vi "Banana Factory.vi"(6 "Strategies.Test":T1, 8 "Clear":bool, 9 "Strategies.Assert":T2, 10 "Peels":refnum<class "BananaPeel.lvclass">[](array[class]), 11 "Variety":string) -> (2 "Bunch":refnum<class "Banana.lvclass">, 3 "Variety Configured":string)   [LabVIEW 2021, in "Bananas.lvlib" / "Banana.lvclass"]
uses:
  Banana.lvclass
  BananaPeel/BananaPeel.lvclass
  Assertion Strategies -- cluster.ctl
  AssertTrue/AssertTrue.lvclass
  AssertFalse/AssertFalse.lvclass
  Test Strategies -- cluster.ctl
  DefineTest/DefineTest.lvclass
  Banana.lvclass/Banana.ctl
  Bananas.lvlib
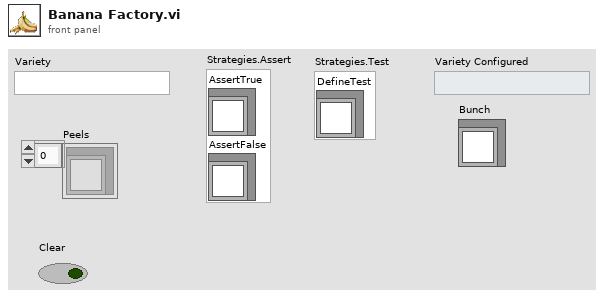
[diagram p1: front panel]
types:
  T1 = typedef "Bananas.lvlib/Test Strategies -- cluster.ctl" = cluster{"DefineTest":refnum<class "DefineTest.lvclass">}
  T2 = typedef "Bananas.lvlib/Assertion Strategies -- cluster.ctl" = cluster{"AssertTrue":refnum<class "AssertTrue.lvclass">, "AssertFalse":refnum<class "AssertFalse.lvclass">}
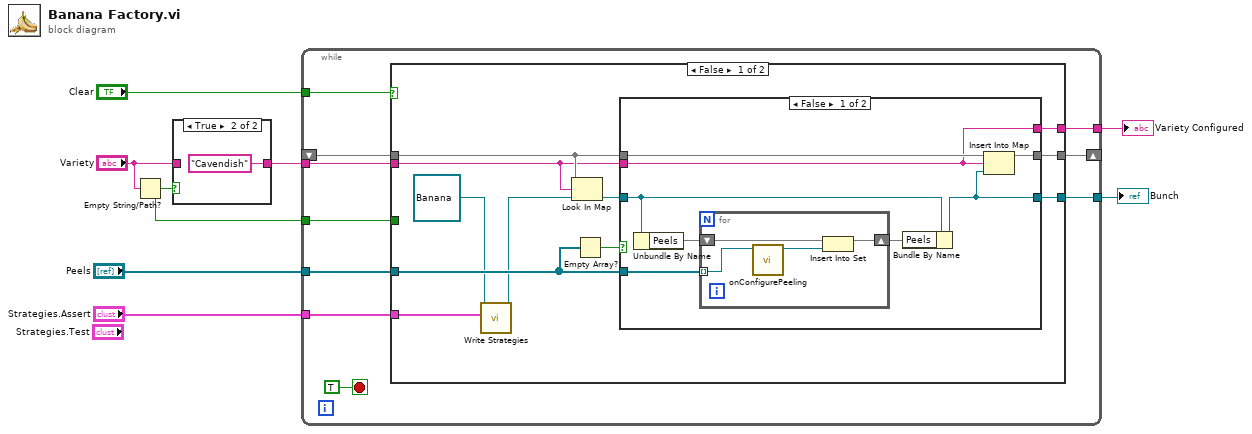
[diagram p0: block diagram]
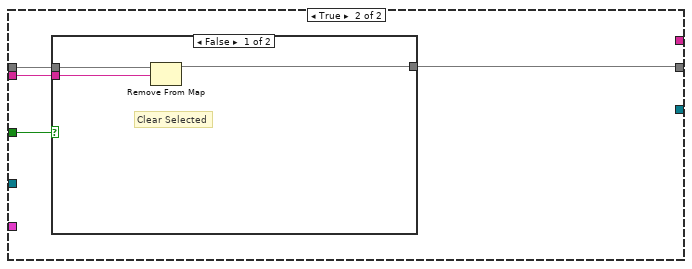
[diagram p4: hidden frame]
diagram:
  n1 = Empty String/Path?(string/path="Variety") -> (empty?=w2:bool)
  n2 = case shown="True" w2 {
    tunnel: [w9 "Cavendish" ("Variety")] -> w7
    tunnel: "Variety" -> [w9 _]
    frame False {
    }
    frame True {
    }
  }
  n3 = while {
    shift-right: [w18] -> _
    shift-left: _ -> [w19]
    tunnel: w7 -> [w16]
    tunnel: [w17] -> w8
    tunnel: "Peels" -> [w15]
    tunnel: "Strategies.Assert" -> [w14]
    tunnel: "Clear" -> [w13]
    tunnel: w2 -> [w12]
    tunnel: [w11] -> w1
    stop <- TRUE stop-if-true
    n4 = case shown="False" w13 {
      tunnel: w19 -> [w31 w49]
      tunnel: [w30 w47] -> w18
      tunnel: [w28 _] -> w17
      tunnel: w16 -> [w27 w48]
      tunnel: w15 -> [w26 _]
      tunnel: w14 -> [w22 _]
      tunnel: w12 -> [_ w50]
      tunnel: [w21 _] -> w11
      frame False {
        n5 = call "Write Strategies.vi"("Strategies.Assert"=w22, "Banana in"=refnum<class "Banana.lvclass"> refnum ("Banana")) -> ("Banana out"=w23:refnum<class "Banana.lvclass">)  [unwired: 9 in]
        n6 = Look In Map(map=w31, key=w27, default value=w23) -> (value=w29:refnum<class "Banana.lvclass">)  [unwired: 1 out]
        n7 = Empty Array?(array=w26) -> (empty?=w25:bool)
        n8 = case shown="False" w25 {
          tunnel: w31 -> [w39 w46]
          tunnel: [w38 w46] -> w30
          tunnel: w29 -> [w34 w45]
          tunnel: [w35 w45] -> w28
          tunnel: w27 -> [w32 w44]
          tunnel: w26 -> [w33 _]
          tunnel: [w32 w44] -> w21
          frame False {
            n9 = Unbundle By Name(w34) -> ("Peels"=w37:set{refnum<class "BananaPeel.lvclass">})
            n10 = for {
              shift-right: [w42] -> w36
              shift-left: w37 -> [w43]
              tunnel: w33 -> [w40] mode=indexing
              n11 = call-dynamic "onConfigurePeeling.vi"("BananaPeel in"=w40) -> ("BananaPeel out"=w41:refnum<class "BananaPeel.lvclass">)  [unwired: 9 in, 1 out]
              n12 = Insert Into Set(10:w41, 11:w43) -> (3:w42:set{refnum<class "BananaPeel.lvclass">})  [unwired: 1 out]
            }
            n13 = Bundle By Name(cluster=w34, "Peels"=w36) -> (w35:refnum<class "Banana.lvclass">)
            n14 = Insert Into Map(map in=w39, key=w32, value=w35) -> (map out=w38:map{string, refnum<class "Banana.lvclass">})  [unwired: 2 out]
          }
          frame True {
          }
        }
      }
      frame True {
        n15 = case shown="False" w50 {
          tunnel: w49 -> [w53 _]
          tunnel: w48 -> [w52 _]
          tunnel: [w51 _] -> w47
          frame False {
            # "Clear Selected"
            n16 = Remove From Map(10:w52, 11:w53) -> (3:w51:map{string, refnum<class "Banana.lvclass">})  [unwired: 2 out]
          }
          frame True {
            # "Clear All"
          }
        }
      }
    }
  }
  "Bunch" <- w8
  "Variety Configured" <- w1
